vi "Komponente Index.vi"(11 "Komponente":T1) -> (3 "Index in Gasliste":i32)   [LabVIEW 2020, in "System Einstellungen V2.lvlib"]
uses:
  System Einstellungen V2.lvlib
  Visualisierungs Elemente/String - Ausgabefeld.ctl
  FT-IR/FGV FT-IR Gasliste Aktionen.ctl
  FT-IR/FT-IR.lvlib
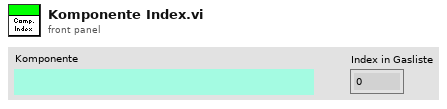
[diagram p1: front panel]
types:
  T1 = typedef "String - Ausgabefeld.ctl" = string
  T2 = typedef "FT-IR.lvlib/FGV FT-IR Gasliste Aktionen.ctl" = enum16{"lesen", "Gasliste FT-IR", "Gasliste ausgelesen", "laden", "speichern", "löschen"}
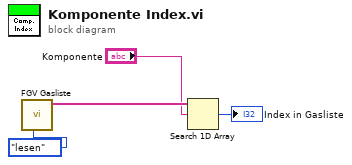
[diagram p0: block diagram]
diagram:
  n1 = call "FGV Gasliste.vi"("Aktionen"=FGV_FT-IR_Gasliste_Aktionen."lesen") -> ("Aktuelle Gasliste FT-IR"=w3:T1[])  [unwired: 8 in, 2 out]
  n2 = Search 1D Array(1D array=w3, element="Komponente") -> (index of element=→"Index in Gasliste":i32)  [unwired: 1 in]
